vi "run-vi-tester.vi"() -> (0 "error out":errorcluster)   [LabVIEW 2014, in "lv-cli-steps.lvlib"]
uses:
  lv-cli-steps.lvlib
  <vilib>/addons/_JKI.lib/_jki_lib_vi_tester_junit_xml_results.llb/TextTestRunner.JUnitXML.lvclass
  <vilib>/Utility/error.llb/DialogType.ctl
  <vilib>/addons/_JKI Toolkits/VI Tester/VI Tester API.llb/Run Tests (Path).vi
  <vilib>/Wiresmith Technology/LabVIEW CLI/CLI Class/CLI.lvclass
  <vilib>/addons/_JKI Toolkits/VI Tester/VI Tester API.llb/VI Tester API.lvlib
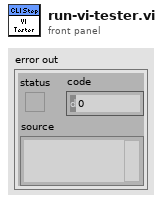
[diagram p1: front panel]
types:
  T1 = typedef "DialogType.ctl" = u16
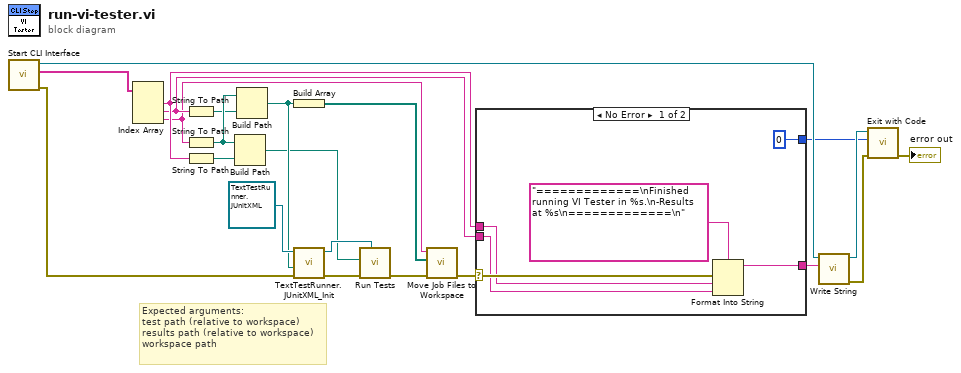
[diagram p0: block diagram]
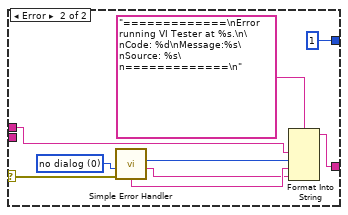
[diagram p2: hidden frame]
diagram:
  # "Expected arguments:\ntest path (relative to workspace)\nresults path (relative to workspace)\nworkspace path"
  n1 = call <vilib>:"Start CLI Interface.vi"() -> ("error out"=w2:errorcluster, "Custom Parameters"=w22:string[], "CLI out"=w18:refnum<class "CLI.lvclass">)  [unwired: 9 in]
  n2 = Index Array(array=w22) -> (element #1=w21:string, element #2=w20:string, element #3=w10:string)  [unwired: 3 in]
  n3 = String To Path(string=w20) -> (path=w12:path)
  n4 = String To Path(string=w10) -> (path=w13:path)
  n5 = String To Path(string=w21) -> (path=w14:path)
  n6 = Build Path(base path=w13, name or relative path=w14) -> (appended path=w3:path)
  n7 = Build Path(base path=w13, name or relative path=w12) -> (appended path=w4:path)
  n8 = Build Array(w4) -> (w11:path[])
  n9 = call <vilib>:"TextTestRunner.JUnitXML_Init.vi"("error in (no error)"=w2, "Report Path"=w4, "TextTestRunner in"=refnum<class "TextTestRunner.JUnitXML.lvclass"> refnum ("TextTestRunner.Ant.lvclass")) -> ("error out"=w5:errorcluster, "TextTestRunner out"=w6:refnum<class "TextTestRunner.JUnitXML.lvclass">)  [unwired: 7 in]
  n10 = call-poly <vilib>:"Run Tests.vi"("TextTestRunner in"=w6, "error in (no error)"=w5, "Test Path"=w3) -> ("error out"=w1:errorcluster)  [unwired: 6 in, 2 out]
  n11 = call "Move Job Files to Workspace.vi"("error in (no error)"=w1, "Generated Files"=w11, "Workspace Path"=w10) -> ("error out"=w9:errorcluster)  [unwired: 8 in]
  n12 = case shown="No Error" w9 {
    selector: w9 -> [w27 w36]
    tunnel: w21 -> [w26 w32]
    tunnel: w20 -> [w25 _]
    tunnel: [w24 w37] -> w19
    tunnel: [0 ("Exit Code (0)") 1 ("Exit Code (0)")] -> w15
    frame No Error {
      n13 = Format Into String(format string="=============\nFinished running VI Tester in %s.\n-Results at %s\n=============\n", error in=w27, w26, w25) -> (resulting string=w24:string)  [unwired: 1 in, 1 out]
    }
    frame Error {
      w35 = T1 0 items=["no dialog", "OK message", "continue or stop message", "OK message + warnings", "continue/stop + warnings"] ("type of dialog (OK msg:1)")
      n14 = call <vilib>:"Simple Error Handler.vi"("type of dialog (OK msg:1)"=w35, "error in (no error)"=w36) -> ("code out"=w29:i32, "source out"=w30:string, "message"=w31:string)  [unwired: 3 in, 2 out]
      n15 = Format Into String(format string="=============\nError running VI Tester at %s.\n\nCode: %d\nMessage:%s\nSource: %s\n=============\n", w32, w29, w31, w30) -> (resulting string=w37:string)  [unwired: 2 in, 1 out]
    }
  }
  n16 = call <vilib>:"Write String.vi"("Text to Write"=w19, "CLI in"=w18) -> ("error out"=w17:errorcluster, "CLI out"=w16:refnum<class "CLI.lvclass">)  [unwired: 8 in]
  n17 = call <vilib>:"Exit with Code.vi"("error in (no error)"=w17, "Exit Code (0)"=w15, "CLI in"=w16) -> ("error out"=→"error out":errorcluster)  [unwired: 8 in]
